vi "UVI_PopUp Menu_Item_Add.vi"(0 "StartIDItem":i32, 5 "PopUpMenuItems":T2(array[cluster]) {"uFlags" items=["MF_STRING"=0, "MF_GRAYED"=1, "MF_DISABLED"=2, "MF_CHECKED"=8, "MF_HILITE"=128, "MF_POPUP"=16, "MF_SEPARATOR"=2048]}, 7 "ParentMenu":string, 11 "error in (no error)":errorcluster) -> (4 "StartIDItem out":i32, 6 "ItemTag":string[](array[string]), 8 "hMenu":u32, 10 "ItemID":i32[](array[numeric]), 15 "error out":errorcluster)   [LabVIEW 2013]
uses:
  TD_PopUp Menu_Flags.ctl
panel:
  in  "VI Refnum":refnum<vi>
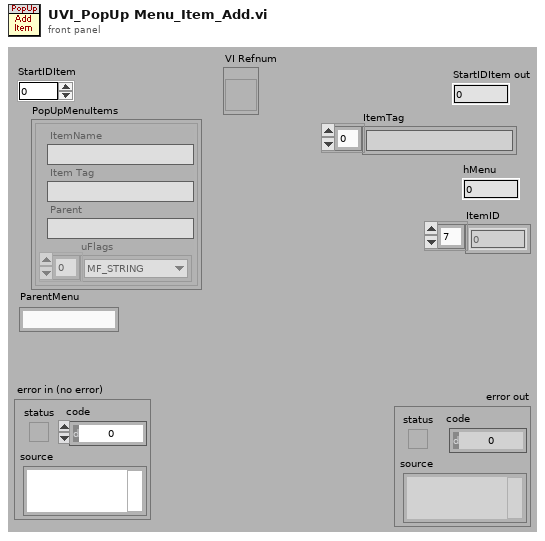
[diagram p1: front panel]
types:
  T1 = typedef "TD_PopUp Menu_Flags.ctl" = u32
  T2 = cluster{"ItemName":string, "Item Tag":string, "Parent":string, "uFlags":T1[]}[]
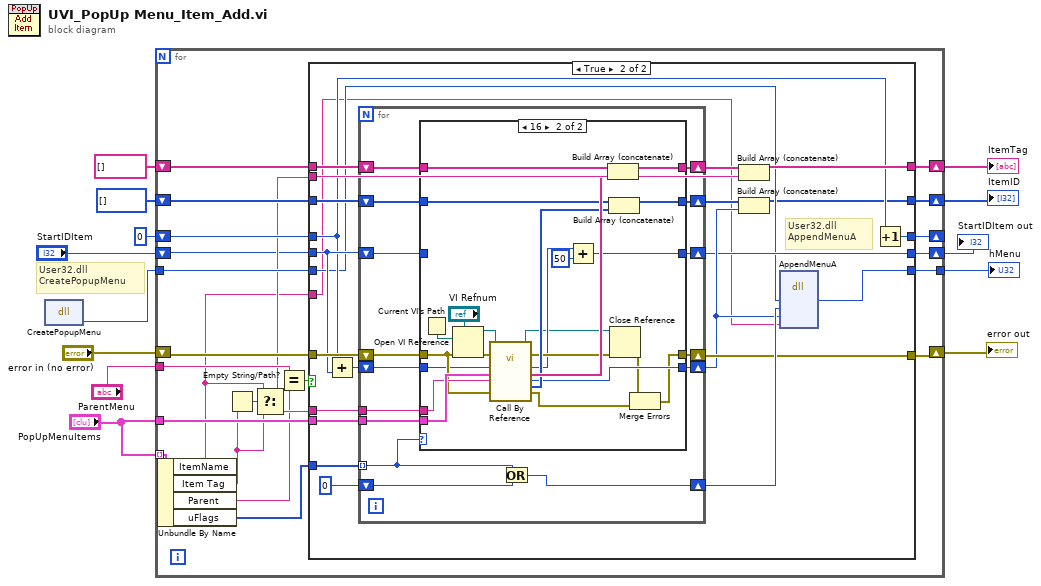
[diagram p0: block diagram]
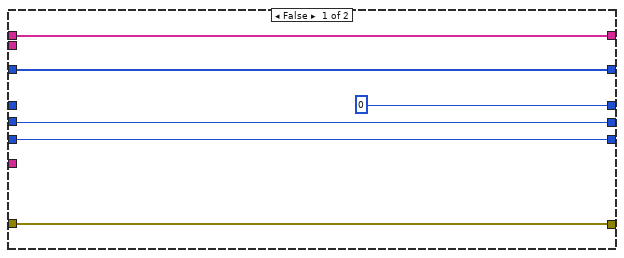
[diagram p2: hidden frame]
diagram:
  # "User32.dll\nCreatePopupMenu"
  n1 = dll-call lib="User32" fn="CreatePopupMenu"() -> (w12:u32)  [unwired: 3 in, 2 out]
  n2 = for {
    tunnel: "PopUpMenuItems" -> [w18] mode=indexing
    tunnel: w12 -> [w35]
    tunnel: [w34] -> w13
    shift-right: [w32] -> _
    shift-left: 0 -> [w33]
    shift-right: [w30] -> w10
    shift-left: string[] [] -> [w31]
    shift-right: [w28] -> w11
    shift-left: i32[] [] -> [w29]
    tunnel: "ParentMenu" -> [w27]
    tunnel: "PopUpMenuItems" -> [w25]
    shift-right: [w23] -> w4
    shift-left: "error in (no error)" -> [w24]
    shift-right: [w19] -> w2
    shift-left: "StartIDItem" -> [w20]
    n3 = Unbundle By Name(w18) -> ("ItemName"=w14:string, "Item Tag"=w15:string, "Parent"=w16:string, "uFlags"=w17:T1[])
    n4 = Empty String/Path?(string/path=w15) -> (empty?=w22:bool)
    n5 = Select(t=w14, s=w22, f=w15) -> (s? t:f=w21:string)
    n6 = Equal?(x=w27, y=w16) -> (x = y?=w26:bool)
    n7 = case shown="True" w26 {
      tunnel: w35 -> [w39 w44]
      tunnel: [w39 w64] -> w34
      tunnel: w17 -> [_ w63]
      tunnel: w14 -> [_ w43]
      tunnel: w20 -> [w37 w46]
      tunnel: w33 -> [_ w45]
      tunnel: [0 w60] -> w32
      tunnel: w31 -> [w41 w57]
      tunnel: w21 -> [_ w48]
      tunnel: [w41 w59] -> w30
      tunnel: w29 -> [w40 w56]
      tunnel: [w40 w42] -> w28
      tunnel: w25 -> [_ w54]
      tunnel: w21 -> [_ w53]
      tunnel: w24 -> [w38 w52]
      tunnel: [w38 w51] -> w23
      tunnel: [w37 w47] -> w19
      frame False {
      }
      frame True {
        # "User32.dll\nAppendMenuA"
        n8 = Add(x=w45, y=w46) -> (x+y=w58:i32)
        n9 = for {
          tunnel: w63 -> [w77] mode=indexing
          shift-right: [w78] -> w61
          shift-left: 0 -> [w79]
          shift-right: [w71] -> w49
          shift-left: w58 -> [w72]
          shift-right: [w73] -> w50
          shift-left: w57 -> [w76]
          shift-right: [w74] -> w55
          shift-left: w56 -> [w75]
          tunnel: w54 -> [w70]
          tunnel: w53 -> [w69]
          shift-right: [w67] -> w51
          shift-left: w52 -> [w68]
          shift-right: [w66] -> w47
          shift-left: w46 -> [w65]
          n10 = case shown="16" w77 {
            tunnel: w76 -> [w83 w107]
            tunnel: w75 -> [w82 w105]
            tunnel: [w82 w103] -> w74
            tunnel: [w83 w102] -> w73
            tunnel: w72 -> [w84 w95]
            tunnel: [w84 w101] -> w71
            tunnel: w70 -> [_ w100]
            tunnel: w69 -> [_ w99]
            tunnel: w68 -> [w81 w98]
            tunnel: [w81 w97] -> w67
            tunnel: [w80 w96] -> w66
            tunnel: w65 -> [w80 _]
            frame 0, Default {
            }
            frame 16 {
              n11 = Current VI's Path() -> (path=w88:path)
              n12 = Open VI Reference(type specifier VI Refnum (for type only)="VI Refnum", vi path=w88, error in (no error)=w98) -> (vi reference=w94:refnum<vi>, error out=w91:errorcluster)  [unwired: 3 out]
              n13 = call-by-ref "?"(reference=w94, error in=w91, "StartIDItem"=w95, "PopUpMenuItems"=w100, "ParentMenu"=w99, "error in (no error)"=w98) -> (reference out=w85:refnum<vi>, error out=w92:errorcluster, "StartIDItem out"=w87:i32, "ItemTag"=w106:string[], "hMenu"=w101:u32, "ItemID"=w104:i32[], 15:"error out"=w89:errorcluster)  [unwired: 7 in]
              n14 = Add(x=w87, y=50) -> (x+y=w96:i32)
              n15 = Build Array (concatenate)(w107, w106) -> (w102:string[])
              n16 = Build Array (concatenate)(w105, w104) -> (w103:u32[])
              n17 = Close Reference(reference=w85, error in (no error)=w92) -> (error out=w90:errorcluster)
              n18 = Merge Errors(w90, w89) -> (w97:errorcluster)
            }
          }
          n19 = Or(x=w77, y=w79) -> (x .or. y?=w78:T1)
        }
        n20 = Build Array (concatenate)(w50, w48) -> (w59:string[])
        n21 = Build Array (concatenate)(w55, w49) -> (w42:u32[])
        n22 = dll-call lib="User32" fn="AppendMenuA"("hMenu"=w44, "wFlags"=w61, "wIDNewItem"=w49, "lpszNewItem"=w43) -> ("hMenu"=w64:u32)  [unwired: 6 in, 3 out]
        n23 = Increment(x=w45) -> (x+1=w60:i32)
      }
    }
  }
  "ItemID" <- w11
  "ItemTag" <- w10
  "hMenu" <- w13
  "error out" <- w4
  "StartIDItem out" <- w2
